vi "FileComparator.vi"() -> ()   [LabVIEW 2009]
panel:
  out "Hash 2":string
  out "Hash 1":string
  in  "Quit":bool
  out "Equal?":bool
  in  "Compare":bool
  in  "File 2":path
  in  "File 1":path
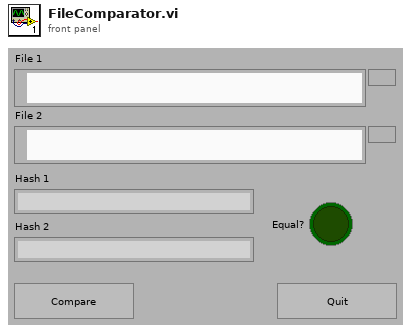
[diagram p1: front panel]
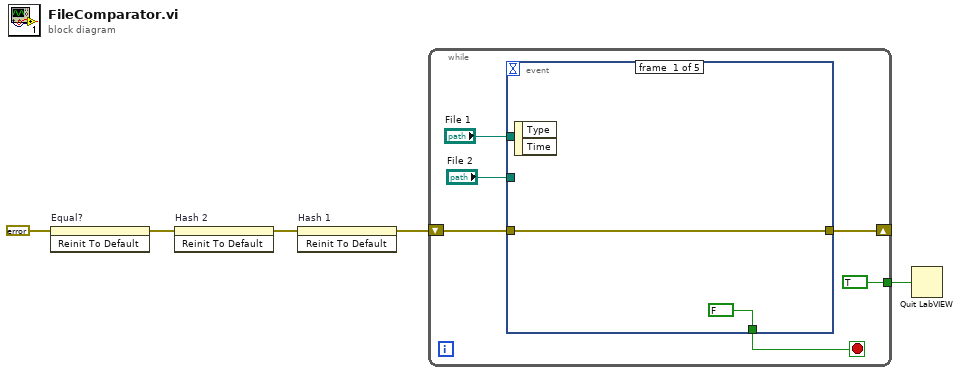
[diagram p0: block diagram]
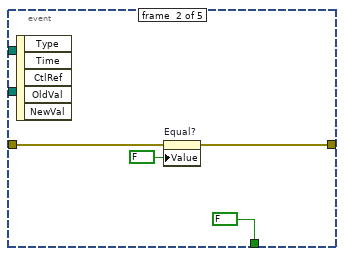
[diagram p2: hidden frame]
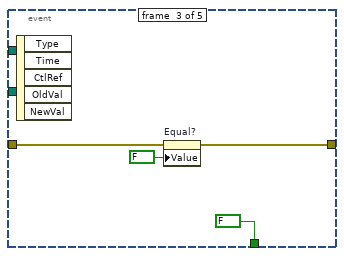
[diagram p3: hidden frame]
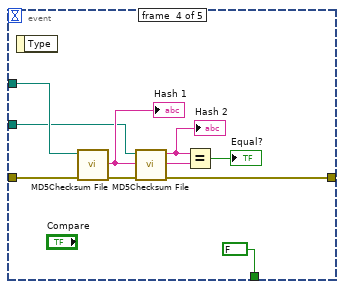
[diagram p4: hidden frame]
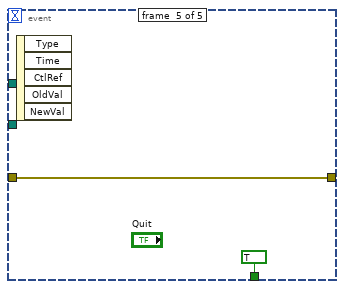
[diagram p5: hidden frame]
diagram:
  n1 = invoke on="Equal?" class="Bool (strict)" method="Reinit To Default"(error in=errorcluster {"status"=FALSE, "code"=0, "source"=""} ("error out")) -> (error out=w3:errorcluster)  [unwired: 2 in, 2 out]
  n2 = invoke on="Hash 2" class="Str" method="Reinit To Default"(error in=w3) -> (error out=w4:errorcluster)  [unwired: 2 in, 2 out]
  n3 = invoke on="Hash 1" class="Str" method="Reinit To Default"(error in=w4) -> (error out=w5:errorcluster)  [unwired: 2 in, 2 out]
  n4 = while {
    shift-right: [w11] -> _
    shift-left: w5 -> [w10]
    tunnel: [TRUE] -> w1
    stop <- w9 stop-if-true
    n5 = event shown="[3] \"Compare\": Value Change" {
      selector: _ -> [_ _ _ _ _]
      dyn-events: _ -> [_ _ _ _ _]
      timeout: _ -> [_ _ _ _ _]
      tunnel: w10 -> [w13 w16 w20 w29 w31]
      tunnel: [w13 w15 w19 w27 w31] -> w11
      tunnel: [FALSE FALSE FALSE FALSE TRUE] -> w9
      tunnel: "File 1" -> [_ _ _ w24 _]
      tunnel: "File 2" -> [_ _ _ w23 _]
      event #0 {
        n6 = event-data() -> ()  [unwired: 1 in, 2 out]
      }
      event #1 {
        n7 = event-data() -> ()  [unwired: 1 in, 5 out]
        n8 = property on="Equal?" class="Bool (strict)"(error in=w16, "Value"=FALSE ("Equal?")) -> (error out=w15:errorcluster)  [unwired: 1 in, 1 out]
      }
      event #2 {
        n9 = event-data() -> ()  [unwired: 1 in, 5 out]
        n10 = property on="Equal?" class="Bool (strict)"(error in=w20, "Value"=FALSE ("Equal?")) -> (error out=w19:errorcluster)  [unwired: 1 in, 1 out]
      }
      event #3 {
        n11 = event-data() -> ()  [unwired: 1 in, 1 out]
        n12 = call <vilib>:"MD5Checksum File.vi"("error in (no error)"=w29, "Path"=w24) -> ("error out"=w28:errorcluster, "MD5 message-digest"=w25:string)  [unwired: 8 in]
        "Hash 1" <- w25
        n13 = call <vilib>:"MD5Checksum File.vi"("error in (no error)"=w28, "Path"=w23) -> ("error out"=w27:errorcluster, "MD5 message-digest"=w22:string)  [unwired: 8 in]
        "Hash 2" <- w22
        n14 = Equal?(x=w22, y=w25) -> (x = y?=→"Equal?":bool)
      }
      event #4 {
        n15 = event-data() -> ()  [unwired: 1 in, 5 out]
      }
    }
  }
  n16 = Quit LabVIEW(quit? (T)=w1) -> ()
